vi "NUMERIC OPERATIONS 2.vi"() -> ()   [LabVIEW 2019]
panel:
  in  "INPUT":dbl
  out "RECIPROCAL":dbl
  out "SQUARE":dbl
  out "SQUAREROOT":dbl
  out "DECREMENT":dbl
  out "INCREMENT":dbl
  # "NUMERIC OPERATIONS 2"
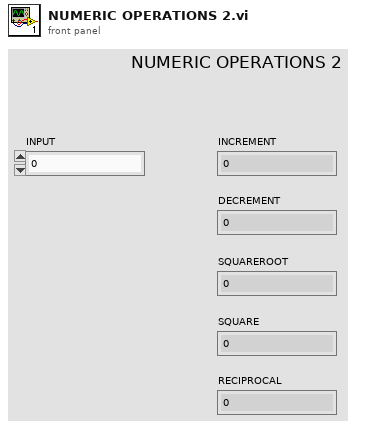
[diagram p1: front panel]
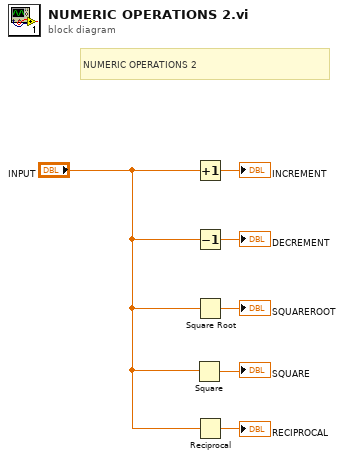
[diagram p0: block diagram]
diagram:
  # "NUMERIC OPERATIONS 2"
  n1 = Square(x="INPUT") -> (x^2=→"SQUARE":dbl)
  n2 = Increment(x="INPUT") -> (x+1=→"INCREMENT":dbl)
  n3 = Decrement(x="INPUT") -> (x-1=→"DECREMENT":dbl)
  n4 = Square Root(x="INPUT") -> (sqrt(x)=→"SQUAREROOT":dbl)
  n5 = Reciprocal(x="INPUT") -> (1/x=→"RECIPROCAL":dbl)
